vi "Update Measurement from Metadata.vi"(6 "default value":variant, 7 "client service_class":string, 8 "error in":errorcluster, 9 "metadata":T1, 10 "run client refnum":refnum<vi>, 11 "file refnums":refnum<vi>[](array[refnum])) -> (0 "error out":errorcluster)   [LabVIEW 2021, in "MeasurementClient Editor.lvlib"]
uses:
  MeasurementClient Editor.lvlib
  <vilib>/gRPC/Generated APIs/ni/measurementlink/measurement/v2/Measurement Service Client V2/RPC Messages/ni_measurementlink_measurement_v2_GetMetadataResponse.ctl
  <vilib>/gRPC/Generated APIs/ni/measurementlink/measurement/v2/Measurement Service Client V2/RPC Messages/ni_measurementlink_measurement_v2_MeasurementDetails.ctl
  <vilib>/gRPC/Generated APIs/ni/measurementlink/measurement/v2/Measurement Service Client V2/RPC Messages/ni_measurementlink_measurement_v2_MeasurementSignature.ctl
  <vilib>/gRPC/Generated APIs/ni/measurementlink/measurement/v2/Measurement Service Client V2/RPC Messages/ni_measurementlink_measurement_v2_ConfigurationParameter.ctl
  <vilib>/gRPC/Generated APIs/ni/measurementlink/measurement/v2/Measurement Service Client V2/RPC Messages/google_protobuf_Field_Kind.ctl
  <vilib>/gRPC/Generated APIs/ni/measurementlink/measurement/v2/Measurement Service Client V2/RPC Messages/ni_measurementlink_measurement_v2_ConfigurationParameter_AnnotationsEntry.ctl
  <vilib>/gRPC/Generated APIs/ni/measurementlink/measurement/v2/Measurement Service Client V2/RPC Messages/google_protobuf_Any.ctl
  <vilib>/gRPC/Generated APIs/ni/measurementlink/measurement/v2/Measurement Service Client V2/RPC Messages/ni_measurementlink_measurement_v2_Output.ctl
  <vilib>/gRPC/Generated APIs/ni/measurementlink/measurement/v2/Measurement Service Client V2/RPC Messages/ni_measurementlink_measurement_v2_Output_AnnotationsEntry.ctl
  <vilib>/gRPC/Generated APIs/ni/measurementlink/measurement/v2/Measurement Service Client V2/RPC Messages/ni_measurementlink_measurement_v2_UserInterfaceDetails.ctl
  <vilib>/Utility/traverseref.llb/TRef TravTarget.ctl
  <vilib>/Utility/traverseref.llb/VI Scripting - Traverse.lvlib
  <vilib>/gRPC/Generated APIs/ni/measurementlink/measurement/v2/Measurement Service Client V2/Measurement Service Client V2.lvlib
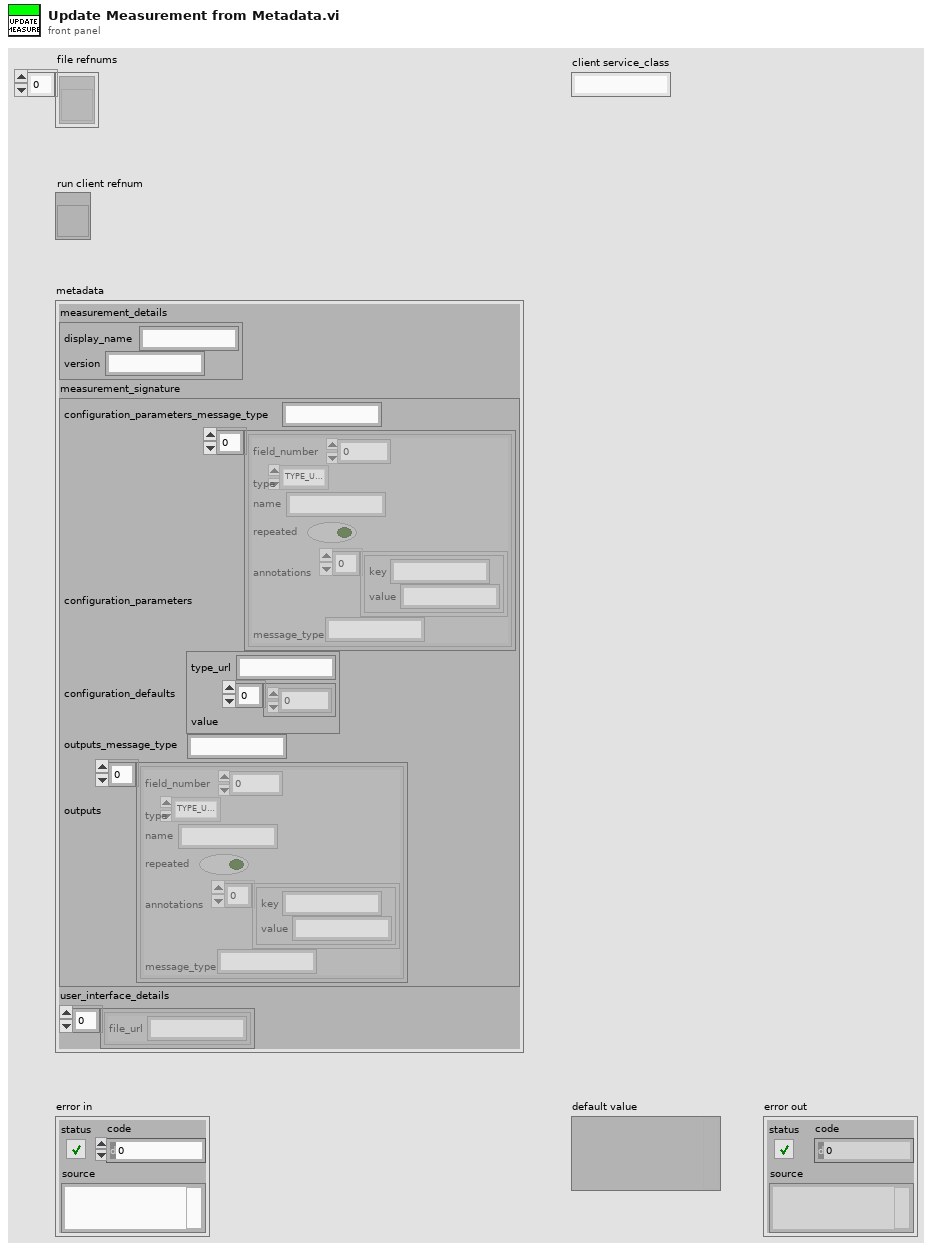
[diagram p1: front panel]
types:
  T1 = typedef "Measurement Service Client V2.lvlib/ni_measurementlink_measurement_v2_GetMetadataResponse.ctl" = cluster{"measurement_details":T2, "measurement_signature":T3, "user_interface_details":T10[]}
  T2 = typedef "Measurement Service Client V2.lvlib/ni_measurementlink_measurement_v2_MeasurementDetails.ctl" = cluster{"display_name":string, "version":string}
  T3 = typedef "Measurement Service Client V2.lvlib/ni_measurementlink_measurement_v2_MeasurementSignature.ctl" = cluster{"configuration_parameters_message_type":string, "configuration_parameters":T4[], "configuration_defaults":T7, "outputs_message_type":string, "outputs":T8[]}
  T4 = typedef "Measurement Service Client V2.lvlib/ni_measurementlink_measurement_v2_ConfigurationParameter.ctl" = cluster{"field_number":i32, "type":T5, "name":string, "repeated":bool, "annotations":T6[], "message_type":string}
  T5 = typedef "Measurement Service Client V2.lvlib/google_protobuf_Field_Kind.ctl" = enum32{"TYPE_UNKNOWN", "TYPE_DOUBLE", "TYPE_FLOAT", "TYPE_INT64", "TYPE_UINT64", "TYPE_INT32", "TYPE_FIXED64", "TYPE_FIXED32", "TYPE_BOOL", "TYPE_STRING", "TYPE_GROUP", "TYPE_MESSAGE", "TYPE_BYTES", "TYPE_UINT32", "TYPE_ENUM", "TYPE_SFIXED32", "TYPE_SFIXED64", "TYPE_SINT32", "TYPE_SINT64"}
  T6 = typedef "Measurement Service Client V2.lvlib/ni_measurementlink_measurement_v2_ConfigurationParameter_AnnotationsEntry.ctl" = cluster{"key":string, "value":string}
  T7 = typedef "Measurement Service Client V2.lvlib/google_protobuf_Any.ctl" = cluster{"type_url":string, "value":u8[]}
  T8 = typedef "Measurement Service Client V2.lvlib/ni_measurementlink_measurement_v2_Output.ctl" = cluster{"field_number":i32, "type":T5, "name":string, "repeated":bool, "annotations":T9[], "message_type":string}
  T9 = typedef "Measurement Service Client V2.lvlib/ni_measurementlink_measurement_v2_Output_AnnotationsEntry.ctl" = cluster{"key":string, "value":string}
  T10 = typedef "Measurement Service Client V2.lvlib/ni_measurementlink_measurement_v2_UserInterfaceDetails.ctl" = cluster{"file_url":string}
  T11 = typedef "TRef TravTarget.ctl" = enum16{"FP", "BD", "Other"}
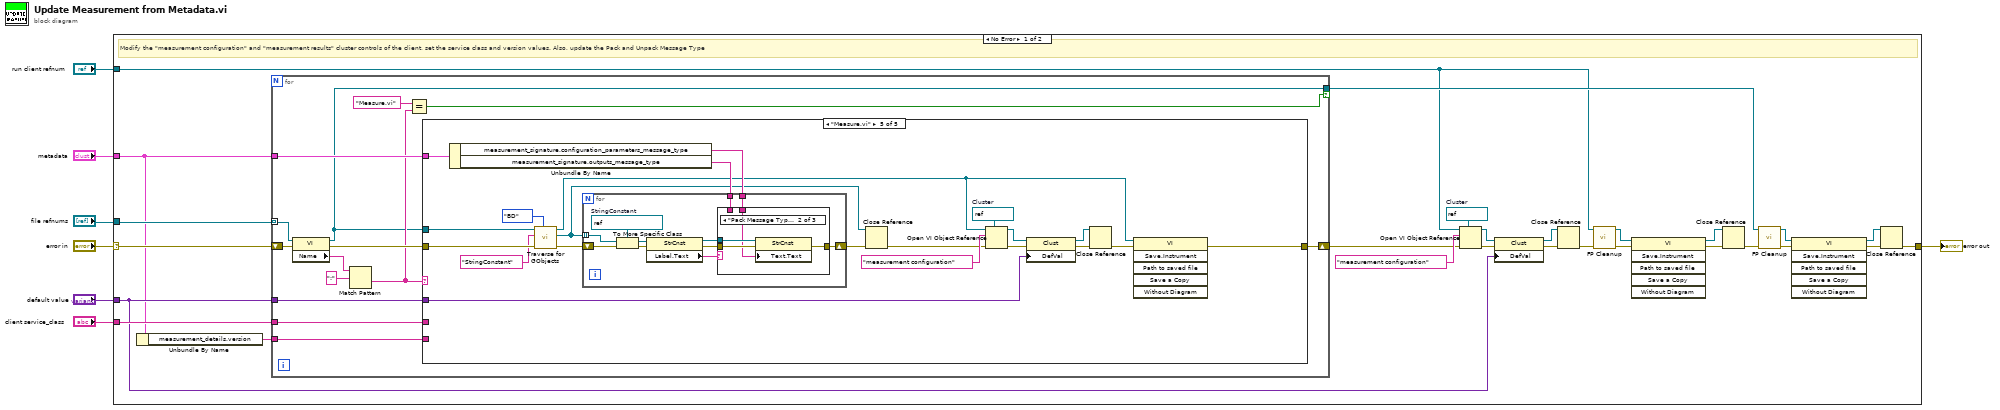
[diagram p0: block diagram]
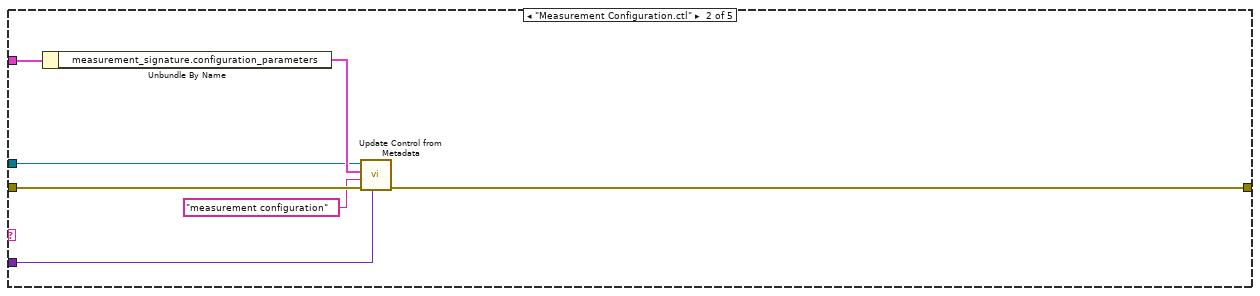
[diagram p3: hidden frame]
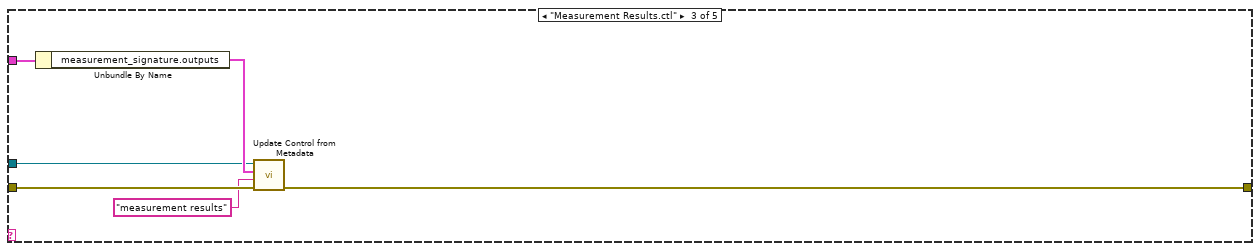
[diagram p4: hidden frame]
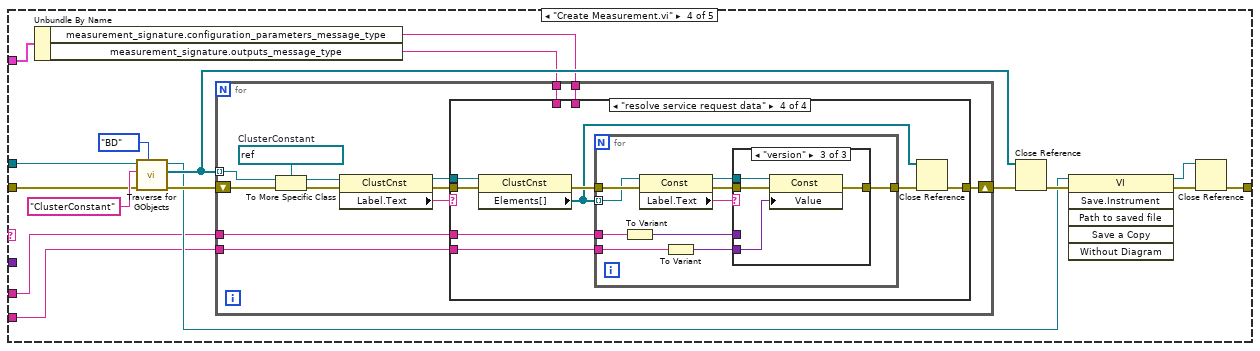
[diagram p5: hidden frame]
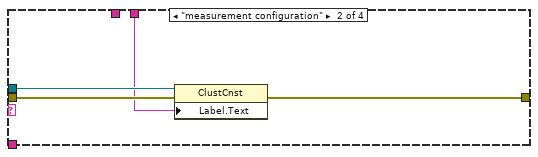
[diagram p7: hidden frame]
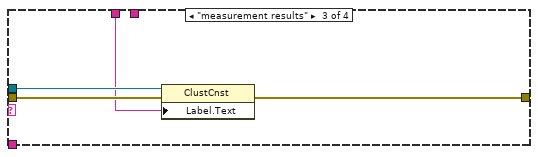
[diagram p8: hidden frame]
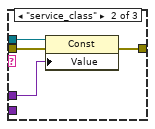
[diagram p10: hidden frame]
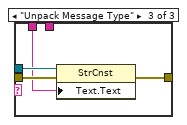
[diagram p12: hidden frame]
diagram:
  n1 = case shown="No Error" "error in" {
    selector: "error in" -> [w33 w169]
    tunnel: [w12 w169] -> w6
    tunnel: "client service_class" -> [w31 _]
    tunnel: "file refnums" -> [w32 _]
    tunnel: "run client refnum" -> [w9 _]
    tunnel: "default value" -> [w19 _]
    tunnel: "metadata" -> [w18 _]
    frame No Error {
      w26 = refnum<vi> refnum  # Cluster
      # "Modify the \"measurement configuration\" and \"measurement results\" cluster controls of the client, set the service class and version values. Also, update the Pack and Unpack Message Type"
      n2 = Unbundle By Name(w18) -> ("measurement_details.version"=w17:string)
      n3 = for {
        shift-right: [w46] -> w21
        shift-left: w33 -> [w47]
        tunnel: w32 -> [w44] mode=indexing
        tunnel: w31 -> [w41]
        tunnel: w19 -> [w40]
        tunnel: w18 -> [w39]
        tunnel: w17 -> [w38]
        tunnel: [w35] -> w15 if=w34
        n4 = property class="VI"(reference=w44, error in=w47) -> (reference out=w35:refnum<vi>, error out=w45:errorcluster, "Name"=w42:string)
        n5 = Match Pattern(string=w42, regular expression=":") -> (after substring=w37:string)  [unwired: 1 in, 3 out]
        n6 = Equal?(x="Measure.vi", y=w37) -> (x = y?=w34:bool)
        n7 = case shown="\"Measure.vi\"" w37 {
          tunnel: w45 -> [w48 w55 w61 w67 w148]
          tunnel: [w48 w51 w57 w76 w147] -> w46
          tunnel: w35 -> [_ w52 w58 w68 w146]
          tunnel: w41 -> [_ _ _ w64 _]
          tunnel: w40 -> [_ w50 _ _ w135]
          tunnel: w39 -> [_ w49 w56 w63 w130]
          tunnel: w38 -> [_ _ _ w62 _]
          frame Default {
          }
          frame "Measurement Configuration.ctl" {
            n8 = Unbundle By Name(w49) -> ("measurement_signature.configuration_parameters"=w53:T4[])
            n9 = call "Update Control from Metadata.vi"("default_value"=w50, "error in"=w55, "control name"="measurement configuration", "parameter data"=w53, "vi refnum"=w52) -> ("error out"=w51:errorcluster)  [unwired: 6 in]
          }
          frame "Measurement Results.ctl" {
            n10 = Unbundle By Name(w56) -> ("measurement_signature.outputs"=w59:T8[])
            n11 = call "Update Control from Metadata.vi"("error in"=w61, "control name"="measurement results", "parameter data"=w59, "vi refnum"=w58) -> ("error out"=w57:errorcluster)  [unwired: 7 in]
          }
          frame "Create Measurement.vi" {
            n12 = Unbundle By Name(w63) -> ("measurement_signature.configuration_parameters_message_type"=w71:string, "measurement_signature.outputs_message_type"=w70:string)
            n13 = call <vilib>:"Traverse for GObjects.vi"("Traverse Target"=TRef_TravTarget."BD", "error in (no error)"=w67, "Class Name"="ClusterConstant", "VI Refnum"=w68) -> ("error out"=w75:errorcluster, "References"=w73:refnum<vi>[], "dup VI Refnum"=w65:refnum<vi>)  [unwired: 4 in, 1 out]
            n14 = for {
              shift-right: [w86] -> w69
              shift-left: w75 -> [w91]
              tunnel: w73 -> [w89] mode=indexing
              tunnel: w71 -> [w84]
              tunnel: w70 -> [w83]
              tunnel: w64 -> [w80]
              tunnel: w62 -> [w79]
              w82 = refnum<vi> refnum  # ClusterConstant
              n15 = To More Specific Class(target class=w82, reference=w89, error in=w91) -> (specific class reference=w88:refnum<vi>, error out=w90:errorcluster)
              n16 = property class="ClustCnst"(reference=w88, error in=w90) -> (reference out=w85:refnum<vi>, error out=w87:errorcluster, "Label.Text"=w81:string)
              n17 = case shown="\"resolve service request data\"" w81 {
                tunnel: [w92 w95 w99 w104] -> w86
                tunnel: w87 -> [w92 w96 w100 w108]
                tunnel: w85 -> [_ w94 w98 w107]
                tunnel: w84 -> [_ w93 _ _]
                tunnel: w83 -> [_ _ w97 _]
                tunnel: w80 -> [_ _ _ w102]
                tunnel: w79 -> [_ _ _ w101]
                frame Default {
                }
                frame "measurement configuration" {
                  n18 = property class="ClustCnst"(reference=w94, error in=w96, "Label.Text"=w93) -> (error out=w95:errorcluster)  [unwired: 1 out]
                }
                frame "measurement results" {
                  n19 = property class="ClustCnst"(reference=w98, error in=w100, "Label.Text"=w97) -> (error out=w99:errorcluster)  [unwired: 1 out]
                }
                frame "resolve service request data" {
                  n20 = property class="ClustCnst"(reference=w107, error in=w108) -> (error out=w106:errorcluster, "Elements[]"=w103:refnum<vi>[])  [unwired: 1 out]
                  n21 = for {
                    tunnel: w103 -> [w117] mode=indexing
                    tunnel: w106 -> [w118]
                    tunnel: [w113] -> w105
                    tunnel: w102 -> [w110]
                    tunnel: w101 -> [w109]
                    n22 = To Variant(anything=w110) -> (Variant=w111:variant)
                    n23 = property class="Const"(reference=w117, error in=w118) -> (reference out=w114:refnum<vi>, error out=w115:errorcluster, "Label.Text"=w116:string)
                    n24 = To Variant(anything=w109) -> (Variant=w112:variant)
                    n25 = case shown="\"version\"" w116 {
                      tunnel: w115 -> [w119 w123 w127]
                      tunnel: w114 -> [_ w122 w126]
                      tunnel: [w119 w121 w125] -> w113
                      tunnel: w112 -> [_ _ w124]
                      tunnel: w111 -> [_ w120 _]
                      frame Default {
                      }
                      frame "service_class" {
                        n26 = property class="Const"(reference=w122, error in=w123, "Value"=w120) -> (error out=w121:errorcluster)  [unwired: 1 out]
                      }
                      frame "version" {
                        n27 = property class="Const"(reference=w126, error in=w127, "Value"=w124) -> (error out=w125:errorcluster)  [unwired: 1 out]
                      }
                    }
                  }
                  n28 = Close Reference(reference=w103, error in (no error)=w105) -> (error out=w104:errorcluster)
                }
              }
            }
            n29 = Close Reference(reference=w73, error in (no error)=w69) -> (error out=w66:errorcluster)
            n30 = invoke class="VI" method="Save.Instrument"(reference=w65, error in=w66) -> (reference out=w78:refnum<vi>, error out=w77:errorcluster)  [unwired: 4 in, 4 out]
            n31 = Close Reference(reference=w78, error in (no error)=w77) -> (error out=w76:errorcluster)
          }
          frame "Measure.vi" {
            w138 = refnum<vi> refnum  # Cluster
            n32 = Unbundle By Name(w130) -> ("measurement_signature.configuration_parameters_message_type"=w141:string, "measurement_signature.outputs_message_type"=w142:string)
            n33 = call <vilib>:"Traverse for GObjects.vi"("Traverse Target"=TRef_TravTarget."BD", "error in (no error)"=w148, "Class Name"="StringConstant", "VI Refnum"=w146) -> ("error out"=w143:errorcluster, "References"=w128:refnum<vi>[], "dup VI Refnum"=w132:refnum<vi>)  [unwired: 4 in, 1 out]
            n34 = for {
              shift-right: [w159] -> w140
              shift-left: w143 -> [w158]
              tunnel: w128 -> [w156] mode=indexing
              tunnel: w142 -> [w150]
              tunnel: w141 -> [w149]
              w155 = refnum<vi> refnum  # StringConstant
              n35 = To More Specific Class(target class=w155, reference=w156, error in=w158) -> (specific class reference=w153:refnum<vi>, error out=w157:errorcluster)
              n36 = property class="StrCnst"(reference=w153, error in=w157) -> (reference out=w152:refnum<vi>, error out=w154:errorcluster, "Label.Text"=w151:string)
              n37 = case shown="\"Pack Message Type\"" w151 {
                tunnel: [w160 w164 w168] -> w159
                tunnel: w154 -> [w160 w163 w167]
                tunnel: w152 -> [_ w162 w166]
                tunnel: w150 -> [_ _ w165]
                tunnel: w149 -> [_ w161 _]
                frame Default {
                }
                frame "Pack Message Type" {
                  n38 = property class="StrCnst"(reference=w162, error in=w163, "Text.Text"=w161) -> (error out=w164:errorcluster)  [unwired: 1 out]
                }
                frame "Unpack Message Type" {
                  n39 = property class="StrCnst"(reference=w166, error in=w167, "Text.Text"=w165) -> (error out=w168:errorcluster)  [unwired: 1 out]
                }
              }
            }
            n40 = Close Reference(reference=w128, error in (no error)=w140) -> (error out=w129:errorcluster)
            n41 = Open VI Object Reference(7:w138, 8:w129, 10:"measurement configuration" ("name/order"), 11:w132) -> (0:w139:errorcluster, 3:w136:refnum<vi>)
            n42 = property class="Clust"(reference=w136, error in=w139, "DefVal"=w135) -> (reference out=w133:refnum<vi>, error out=w137:errorcluster)
            n43 = Close Reference(reference=w133, error in (no error)=w137) -> (error out=w134:errorcluster)
            n44 = invoke class="VI" method="Save.Instrument"(reference=w132, error in=w134) -> (error out=w147:errorcluster)  [unwired: 4 in, 5 out]
          }
        }
      }
      n45 = Open VI Object Reference(7:w26, 8:w21, 10:"measurement configuration" ("name/order"), 11:w9) -> (0:w27:errorcluster, 3:w24:refnum<vi>)
      n46 = property class="Clust"(reference=w24, error in=w27, "DefVal"=w19) -> (reference out=w23:refnum<vi>, error out=w25:errorcluster)
      n47 = Close Reference(reference=w23, error in (no error)=w25) -> (error out=w20:errorcluster)
      n48 = call "FP Cleanup.vi"("error in"=w20, "vi refnum"=w9) -> ("error out"=w10:errorcluster, "vi refnum out"=w8:refnum<vi>)  [unwired: 8 in]
      n49 = invoke class="VI" method="Save.Instrument"(reference=w8, error in=w10) -> (reference out=w29:refnum<vi>, error out=w28:errorcluster)  [unwired: 4 in, 4 out]
      n50 = Close Reference(reference=w29, error in (no error)=w28) -> (error out=w30:errorcluster)
      n51 = call "FP Cleanup.vi"("error in"=w30, "vi refnum"=w15) -> ("error out"=w16:errorcluster, "vi refnum out"=w13:refnum<vi>)  [unwired: 8 in]
      n52 = invoke class="VI" method="Save.Instrument"(reference=w13, error in=w16) -> (reference out=w11:refnum<vi>, error out=w14:errorcluster)  [unwired: 4 in, 4 out]
      n53 = Close Reference(reference=w11, error in (no error)=w14) -> (error out=w12:errorcluster)
    }
    frame Error {
      # "Pass"
    }
  }
  "error out" <- w6
